vi "Save TIFF.vi"(8 "error in (no error)":errorcluster, 10 "Path":path, 11 "ImageHandler in":refnum<class "ImageHandler.lvclass">) -> (0 "error out":errorcluster, 3 "ImageHandler out":refnum<class "ImageHandler.lvclass">)   [LabVIEW 2022 SP3, in "ImageHandler.lvlib" / "ImageHandler.lvclass"]
uses:
  ImageHandler.lvclass
  ImageHandler.lvclass/ImageHandler.ctl
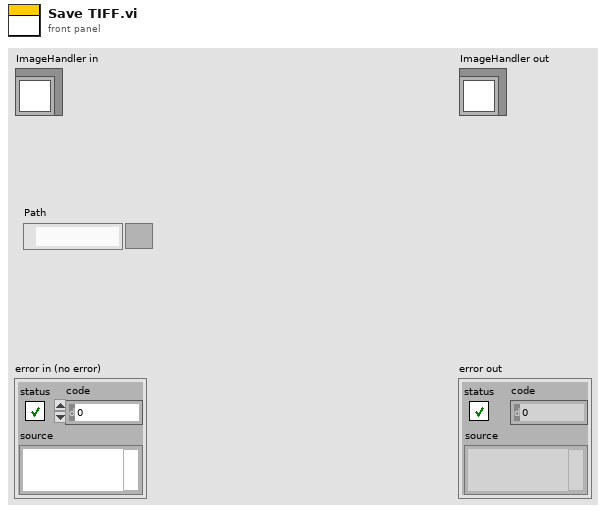
[diagram p1: front panel]
types:
  T1 = typedef "IMAQ Image.ctl" = refnum<image>
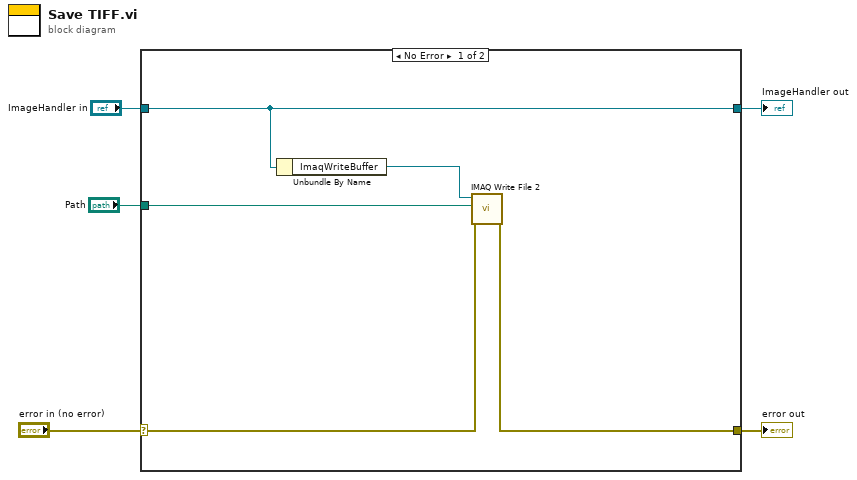
[diagram p0: block diagram]
diagram:
  n1 = case shown="No Error" "error in (no error)" {
    selector: "error in (no error)" -> [w8 w12]
    tunnel: [w7 w12] -> w4
    tunnel: [w10 w11] -> w2
    tunnel: "ImageHandler in" -> [w10 w11]
    tunnel: "Path" -> [w6 _]
    frame No Error {
      n2 = Unbundle By Name(w10) -> ("ImaqWriteBuffer"=w9:T1)
      n3 = call-poly "IMAQ Write File 2"("error in (no error)"=w8, "File Path"=w6, "Image"=w9) -> ("error out"=w7:errorcluster)  [unwired: 7 in, 1 out]
    }
    frame Error {
    }
  }
  "error out" <- w4
  "ImageHandler out" <- w2
